vi "Meta Data to TDMS.vi"(6 "Channel name":string, 7 "Group name":string, 8 "Error In":errorcluster, 9 "Name":string, 10 "Value":variant, 11 "tdms file":refnum<k34>) -> (0 "Error Out":errorcluster, 3 "tdms file out":refnum<k34>)   [LabVIEW 2016]
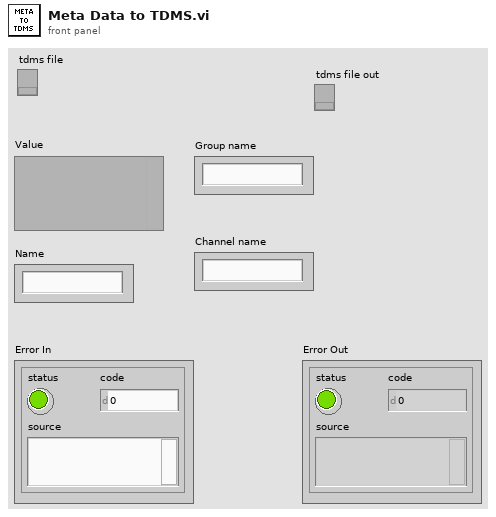
[diagram p1: front panel]
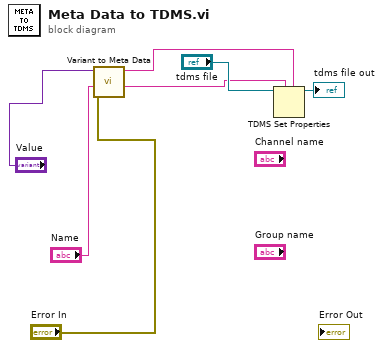
[diagram p0: block diagram]
diagram:
  n1 = call "Variant to Meta Data.vi"("Error In"="Error In", "Name"="Name", "Value"="Value") -> ("Name out"=w1:string, "Meta data"=w2:string)  [unwired: 5 in, 2 out]
  n2 = TDMS Set Properties(5:w2, 7:w1, 11:"tdms file") -> (3:→"tdms file out":refnum<k34>)  [unwired: 3 in, 3 out]
